vi "Save Data I16.vi"(8 "error in (no error)":errorcluster, 10 "Data":i16[][](array[numeric]), 11 "Pulse Driver in":refnum<class "Pulse Driver.lvclass">) -> (0 "error out":errorcluster, 3 "Pulse Driver out":refnum<class "Pulse Driver.lvclass">)   [LabVIEW 2016, in "Pulse Driver.lvclass"]
uses:
  Pulse Driver.lvclass
  C:/github/NHMFL_Core/Libraries/Instruments/Instrument Driver/Instrument Driver.lvclass
  Pulse Driver.lvclass/Pulse Driver.ctl
  Instrument Driver/Instrument Driver.lvclass/Instrument Driver.ctl
  Read tdms file.vi
  Instrument Driver/Read Group name.vi
  Instrument Driver/Read Channel names.vi
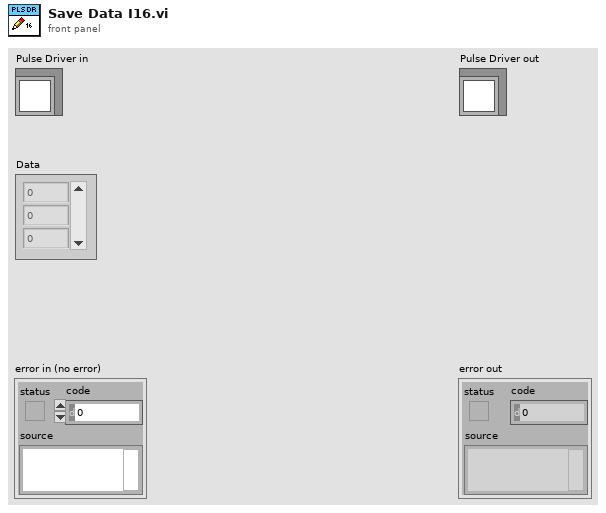
[diagram p1: front panel]
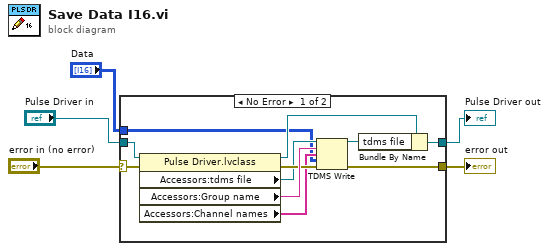
[diagram p0: block diagram]
diagram:
  n1 = case shown="No Error" "error in (no error)" {
    selector: "error in (no error)" -> [w6 w18]
    tunnel: [w7 w18] -> w4
    tunnel: [w8 w17] -> w2
    tunnel: "Pulse Driver in" -> [w9 w17]
    tunnel: "Data" -> [w10 _]
    frame No Error {
      n2 = property class="Pulse Driver.lvclass"(reference=w9, error in=w6) -> (reference out=w12:refnum<class "Pulse Driver.lvclass">, error out=w15:errorcluster, "Accessors:tdms file"=w13:refnum<k34>, "Accessors:Group name"=w16:string, "Accessors:Channel names"=w14:string[])
      n3 = TDMS Write(0:w13, 5:w16, 7:w14, 9:w10, 11:w15) -> (4:w11:refnum<k34>, 15:w7:errorcluster)  [unwired: 1 in, 2 out]
      n4 = Bundle By Name(cluster=w12, "tdms file"=w11) -> (w8:refnum<class "Pulse Driver.lvclass">)
    }
    frame Error {
    }
  }
  "error out" <- w4
  "Pulse Driver out" <- w2
